vi "Read Message (TCP).vi"(6 "prev data info":T1, 8 "error in":errorcluster, 9 "options":T2={"ignore timeout error"=TRUE, "timeout ms (1000)"=1000}, 11 "connection info in":T4) -> (0 "error out":errorcluster, 1 "name":T3, 2 "data string":string, 3 "connection info out":T4, 4 "data info":T1, 5 "timed out":bool)   [LabVIEW 2013, in "NI STM.lvlib"]
doc: "This VI reads an incoming package of data from a host. This VI parses the package and extracts the data name and type as described in the meta data.\n\nFor the package to be parsed correctly, the meta data must be consistent in both the sender and the receiver. The data is packaged based on the existing meta data on the sender. \n\nUse the \"STM Read Meta Data\" and \"STM Write Meta Data\" VIs to ensure that both client and server have the same meta data.\n\nThe data is returned as a string. It is the responsibility of the user to cast it to the appropriate type."
uses:
  NI STM.lvlib
  TCP Connection Info.ctl
  SubVIs/MetaDataElement.ctl
  TCP Read Options.ctl
  TCP Data Info.ctl
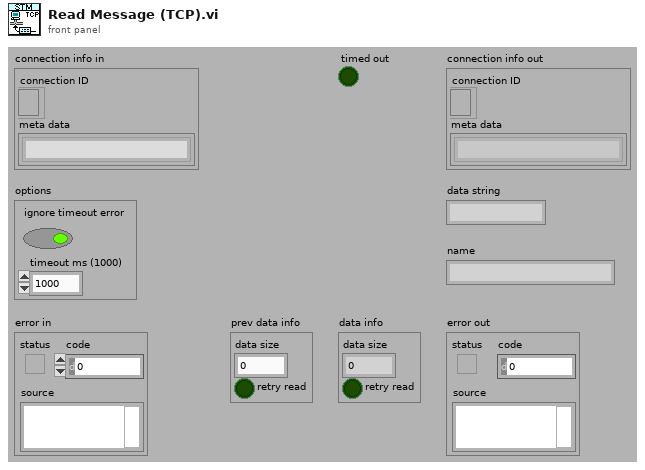
[diagram p1: front panel]
types:
  T1 = typedef "NI STM.lvlib/TCP Data Info.ctl" = cluster{"data size":i32, "retry read":bool}
  T2 = typedef "NI STM.lvlib/TCP Read Options.ctl" = cluster{"ignore timeout error":bool, "timeout ms (1000)":i32}
  T3 = typedef "NI STM.lvlib/MetaDataElement.ctl" = string
  T4 = typedef "NI STM.lvlib/TCP Connection Info.ctl" = cluster{"connection ID":refnum<k5>, "meta data":T3[]}
  T5 = enum16{"Standard", "Buffered", "CRLF", "Immediate"}
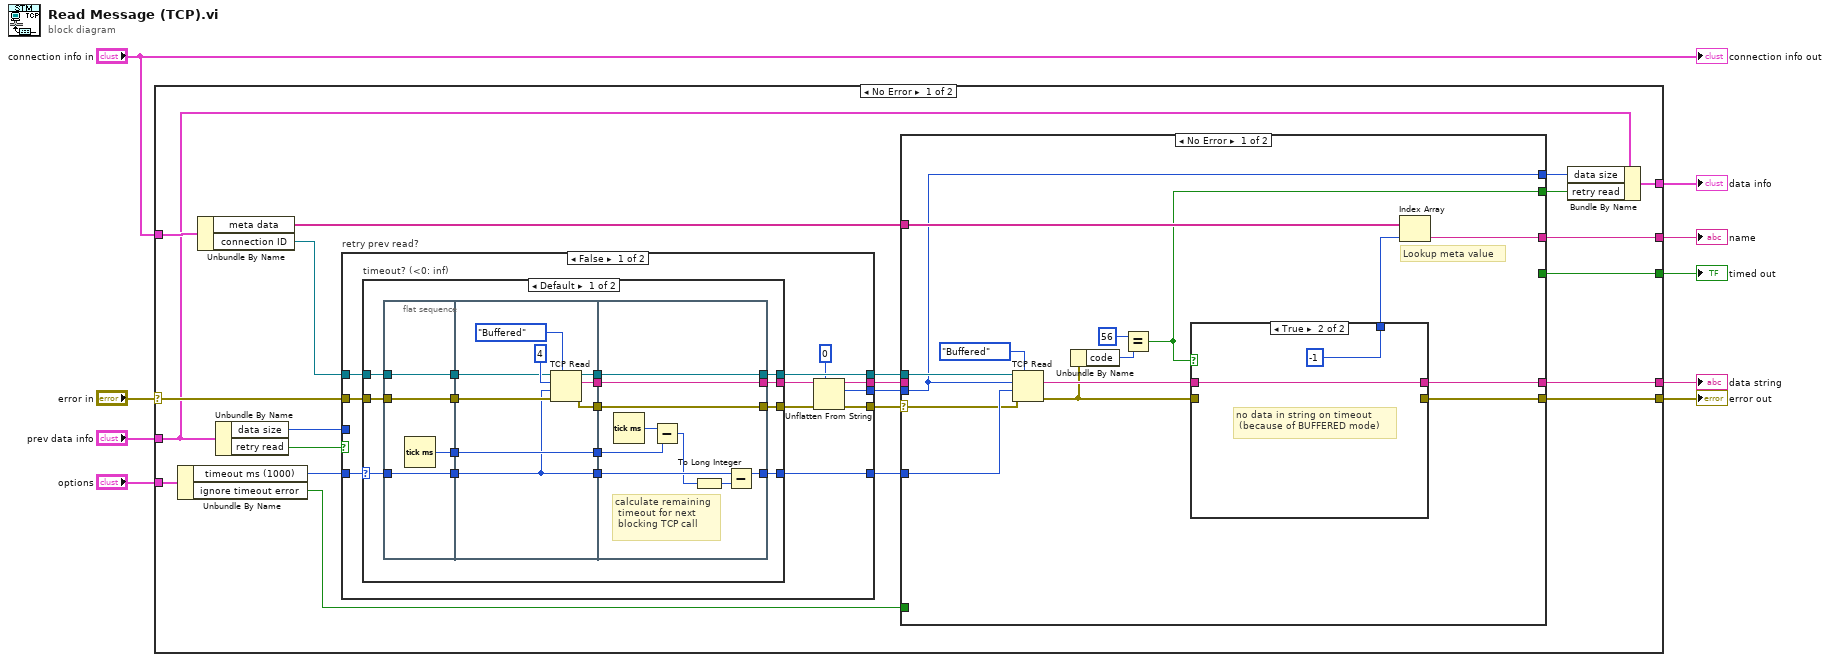
[diagram p0: block diagram]
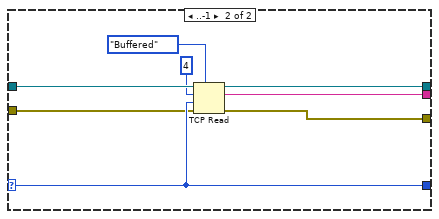
[diagram p2: hidden frame]
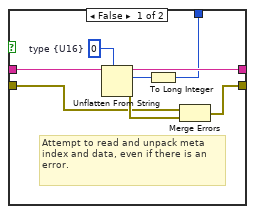
[diagram p4: hidden frame]
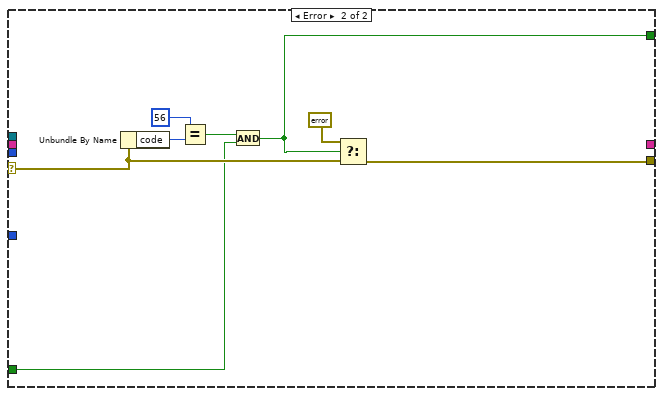
[diagram p5: hidden frame]
diagram:
  n1 = case shown="No Error" "error in" {
    selector: "error in" -> [w22 w126]
    tunnel: "connection info in" -> [w21 _]
    tunnel: [w29 w126] -> w9
    tunnel: [w28 _] -> w8
    tunnel: [w27 _] -> w7
    tunnel: [w11 _] -> w4
    tunnel: "options" -> [w23 _]
    tunnel: "prev data info" -> [w12 _]
    tunnel: [w10 _] -> w1
    frame No Error {
      n2 = Unbundle By Name(w23) -> ("timeout ms (1000)"=w20:i32, "ignore timeout error"=w26:bool)
      n3 = Unbundle By Name(w21) -> ("meta data"=w24:T3[], "connection ID"=w25:refnum<k5>)
      n4 = Unbundle By Name(w12) -> ("data size"=w15:i32, "retry read"=w16:bool)
      n5 = case "retry prev read?" shown="False" w16 {
        tunnel: [w34 _] -> w31
        tunnel: [w42 w91] -> w30
        tunnel: [w33 w92] -> w18
        tunnel: w25 -> [w41 w91]
        tunnel: w22 -> [w40 w92]
        tunnel: w20 -> [w39 w90]
        tunnel: [w38 w90] -> w19
        tunnel: [w32 w89] -> w17
        tunnel: w15 -> [_ w89]
        frame False {
          n6 = case "timeout? (<0: inf)" shown="Default" w39 {
            selector: w39 -> [w43 w88]
            tunnel: [w49 w87] -> w35
            tunnel: [w48 w86] -> w42
            tunnel: [w47 w85] -> w36
            tunnel: w41 -> [w46 w84]
            tunnel: w40 -> [w45 w83]
            tunnel: [w44 w88] -> w38
            frame Default {
              n7 = flat-sequence {
                tunnel: w45 -> [w61]
                tunnel: w46 -> [w62]
                tunnel: [w62] -> w58
                tunnel: [w61] -> w57
                tunnel: [w60] -> w56
                tunnel: [w59] -> w55
                tunnel: w43 -> [w59]
                tunnel: [w70] -> w54
                tunnel: [w69] -> w53
                tunnel: [w68] -> w52
                tunnel: w58 -> [w67]
                tunnel: w57 -> [w66]
                tunnel: [w65] -> w51
                tunnel: w56 -> [w65]
                tunnel: w55 -> [w64]
                tunnel: [w64] -> w50
                tunnel: [w78] -> w47
                tunnel: [w79] -> w48
                tunnel: [w80] -> w49
                tunnel: w54 -> [w80]
                tunnel: w53 -> [w79]
                tunnel: w52 -> [w78]
                tunnel: w51 -> [w76]
                tunnel: w50 -> [w75]
                tunnel: [w73] -> w44
                frame #0 {
                  n8 = Tick Count (ms)() -> (millisecond timer value=w60:u32)
                }
                frame #1 {
                  n9 = TCP Read(connection ID=w67, bytes to read=4, error in (no error)=w66, 7:T5."Buffered" ("mode (standard)"), 9:w64) -> (connection ID out=w69:refnum<k5>, data out=w70:string, error out=w68:errorcluster)
                }
                frame #2 {
                  # "calculate remaining\n timeout for next\n blocking TCP call"
                  n10 = Tick Count (ms)() -> (millisecond timer value=w77:u32)
                  n11 = Subtract(x=w77, y=w76) -> (x-y=w74:u32)
                  n12 = To Long Integer(number=w74) -> (32bit integer=w72:i32)
                  n13 = Subtract(x=w75, y=w72) -> (x-y=w73:i32)
                }
              }
            }
            frame ..-1 {
              n14 = TCP Read(connection ID=w84, bytes to read=4, error in (no error)=w83, 7:T5."Buffered" ("mode (standard)"), 9:w88) -> (connection ID out=w86:refnum<k5>, data out=w87:string, error out=w85:errorcluster)
            }
          }
          n15 = Unflatten From String(type=0 ("bytes to read"), binary string=w35, error in (no error)=w36) -> (rest of the binary string=w34:string, value=w32:i32, error out=w33:errorcluster)  [unwired: 1 in, 1 out]
        }
        frame True {
          # "previous read timed out while trying to pop data off byte stream.\n skip \"read header\" in this call of VI and just do \"read data\" again\n with previous read's data size."
        }
      }
      n16 = case shown="No Error" w18 {
        selector: w18 -> [w94 w125]
        tunnel: w31 -> [_ _]
        tunnel: w30 -> [w107 _]
        tunnel: w24 -> [w106 _]
        tunnel: [w97 w124] -> w29
        tunnel: w26 -> [_ w122]
        tunnel: [w99 _] -> w13
        tunnel: [w105 _] -> w28
        tunnel: [w103 _] -> w27
        tunnel: w19 -> [w101 _]
        tunnel: w17 -> [w93 _]
        tunnel: [w93 _] -> w14
        tunnel: [_ w118] -> w10
        frame No Error {
          # "Lookup meta value"
          n17 = TCP Read(connection ID=w107, bytes to read=w93, error in (no error)=w94, 7:T5."Buffered" ("mode (standard)"), 9:w101) -> (data out=w104:string, error out=w98:errorcluster)  [unwired: 1 out]
          n18 = Unbundle By Name(w98) -> ("code"=w102:i32)
          n19 = Equal?(x=56 ("code"), y=w102) -> (x = y?=w99:bool)
          n20 = case shown="True" w99 {
            tunnel: w104 -> [w115 w117]
            tunnel: [w113 w117] -> w103
            tunnel: [w108 -1 ("type {U16}")] -> w96
            tunnel: w98 -> [w109 _]
            tunnel: [w111 _] -> w97
            frame False {
              w114 = u16 0  # type {U16}
              # "Attempt to read and unpack meta index and data, even if there is an error."
              n21 = Unflatten From String(type=w114, binary string=w115) -> (rest of the binary string=w113:string, value=w112:u16, error out=w110:errorcluster)  [unwired: 1 in, 2 out]
              n22 = To Long Integer(number=w112) -> (32bit integer=w108:i32)
              n23 = Merge Errors(w109, w110) -> (w111:errorcluster)
            }
            frame True {
              # "no data in string on timeout\n (because of BUFFERED mode)"
            }
          }
          n24 = Index Array(array=w106, index=w96) -> (element=w105:T3)
        }
        frame Error {
          n25 = Unbundle By Name(w125) -> ("code"=w123:i32)
          n26 = Equal?(x=56 ("code"), y=w123) -> (x = y?=w120:bool)
          n27 = And(x=w120, y=w122) -> (x .and. y?=w118:bool)
          n28 = Select(t=errorcluster {"status"=FALSE, "code"=0, "source"=""} ("error out"), s=w118, f=w125) -> (s? t:f=w124:errorcluster)
        }
      }
      n29 = Bundle By Name(cluster=w12, "data size"=w14, "retry read"=w13) -> (w11:T1)
    }
    frame Error {
    }
  }
  "error out" <- w9
  "data string" <- w7
  "name" <- w8
  "data info" <- w4
  "timed out" <- w1
  "connection info out" <- "connection info in"
